vi "Introspection Core.vi"(8 "error in (no error)":errorcluster, 11 "TestLNA in":refnum<class "TestLNA.lvclass">) -> (0 "error out":errorcluster, 2 "CS++Messages":refnum<class "Message.lvclass">[](array[class]), 3 "TestLNA out":refnum<class "TestLNA.lvclass">)   [LabVIEW 2014, in "TestLNA.lvlib" / "TestLNA.lvclass"]
doc: "This vi delivers a list with all messages this actor reacts to. \n\nNote that all inherited classes have to overwrite it."
uses:
  TestLNA.lvclass
  CSPP_Core/Actors/CS++BaseActor/CS++BaseActor.lvclass
  LNA Messages/LNA Connection Status Msg/LNA Connection Status Msg.lvclass
  LNA Messages/LNA Return Message Msg/LNA Return Message Msg.lvclass
  Test LNA Messages/Number Msg/Number Msg.lvclass
  Test LNA Messages/Ping Msg/Ping Msg.lvclass
  Test LNA Messages/Remote Message Msg/Remote Message Msg.lvclass
  <vilib>/ActorFramework/Message/Message.lvclass
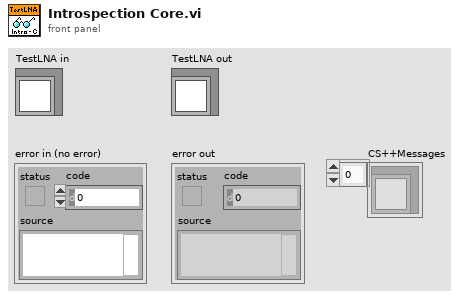
[diagram p1: front panel]
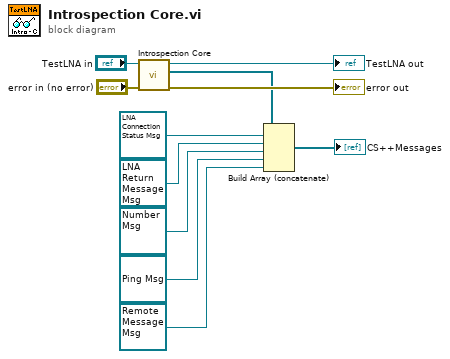
[diagram p0: block diagram]
diagram:
  n1 = call-parent "Introspection Core.vi"("error in (no error)"="error in (no error)", "CS++BaseActor in"="TestLNA in") -> ("error out"=→"error out":errorcluster, "CS++Messages"=w10:refnum<class "Message.lvclass">[], "CS++BaseActor out"=→"TestLNA out":refnum<class "TestLNA.lvclass">)  [unwired: 7 in]
  n2 = Build Array (concatenate)(w10, refnum<class "LNA Connection Status Msg.lvclass"> refnum ("TestLNA.lvlib:LNA Connection Status Msg.lvclass"), refnum<class "LNA Return Message Msg.lvclass"> refnum ("TestLNA.lvlib:LNA Return Message Msg.lvclass"), refnum<class "Number Msg.lvclass"> refnum ("TestLNA.lvlib:Number Msg.lvclass"), refnum<class "Ping Msg.lvclass"> refnum ("TestLNA.lvlib:Ping Msg.lvclass"), refnum<class "Remote Message Msg.lvclass"> refnum ("TestLNA.lvlib:Remote Message Msg.lvclass")) -> (→"CS++Messages":refnum<class "Message.lvclass">[])
